vi "visualizeTDMS.vi"(8 "错误输入（无错误）":errorcluster) -> (0 "错误输出":errorcluster, 2 "强度图":dbl[][](graph), 3 "数据采集时间":string="2016/1/11 16:05:34")   [LabVIEW 2013]
panel:
  in  "save excel":bool
  out "file path out":path
  out "大小":i32
  out "数值":i32
  in  "确定按钮":bool
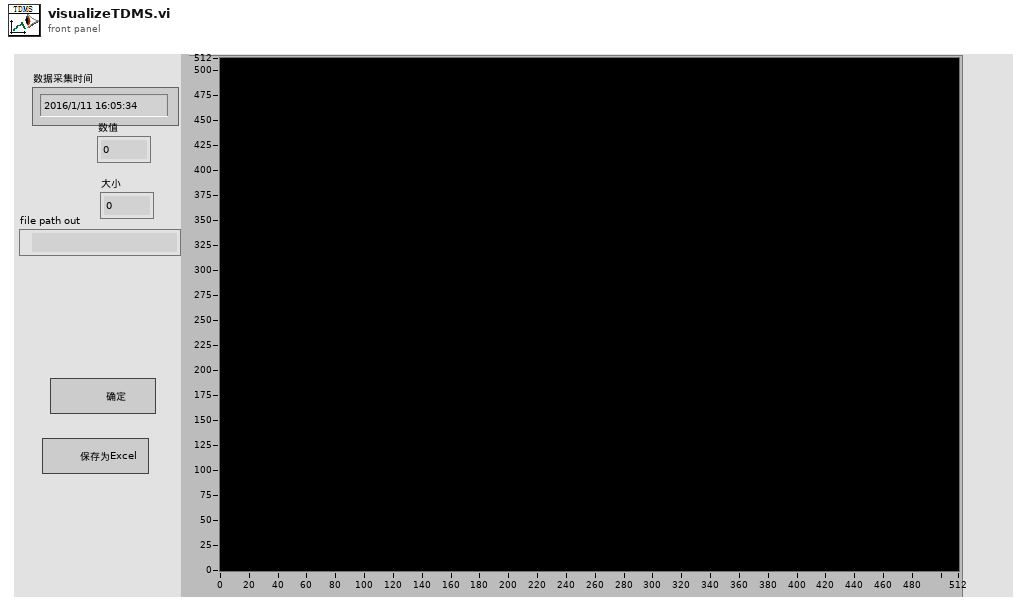
[diagram p1: front panel]
types:
  T1 = cluster{"Vx_Max":dbl, "Vy_Max":dbl, "Tx":dbl, "Row_N":i32, "Ratio":dbl}
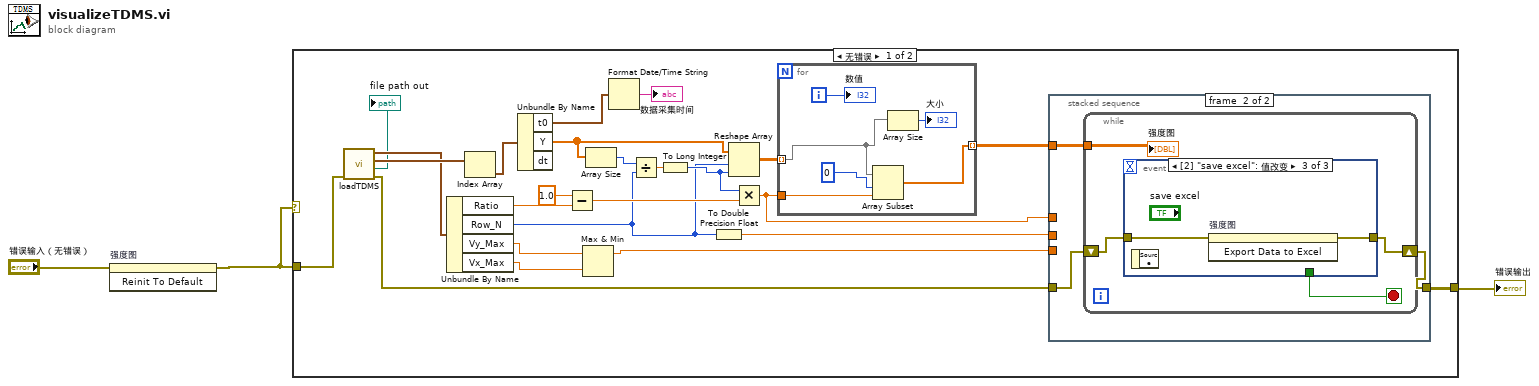
[diagram p0: block diagram]
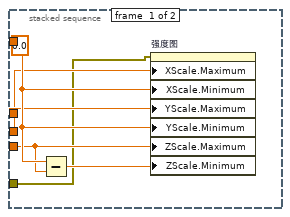
[diagram p2: hidden frame]
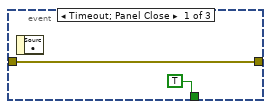
[diagram p3: hidden frame]
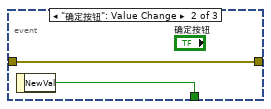
[diagram p4: hidden frame]
diagram:
  n1 = invoke on="强度图" class="IntGraph (严格)" method="Reinit To Default"(error in="错误输入（无错误）") -> (error out=w1:errorcluster)  [unwired: 2 in, 2 out]
  n2 = case shown="无错误" w1 {
    tunnel: w1 -> [w18 w53]
    tunnel: [w16 w53] -> w3
    frame No Error {
      n3 = call "loadTDMS.vi"("错误输入（无错误）"=w18) -> ("错误输出"=w17:errorcluster, "file path out"=→"file path out":path, "数据"=w27:waveform(dbl)[], "输出簇"=w15:T1)  [unwired: 7 in]
      n4 = Unbundle By Name(w15) -> ("Ratio"=w13:dbl, "Row_N"=w6:i32, "Vy_Max"=w21:dbl, "Vx_Max"=w20:dbl)
      n5 = Index Array(array=w27) -> (element=w26:waveform(dbl))  [unwired: 1 in]
      n6 = Unbundle By Name(w26) -> ("t0"=w25:timestamp, "Y"=w22:dbl[])  [unwired: 1 out]
      n7 = Subtract(x=1.0, y=w13) -> (x-y=w9:dbl)
      n8 = Max & Min(x=w21, y=w20) -> (max(x,y)=w19:dbl)  [unwired: 1 out]
      n9 = Array Size(array=w22) -> (size(s)=w23:i32)
      n10 = Format Date/Time String(seconds (now)=w25) -> (date/time string=→"数据采集时间":string)  [unwired: 2 in]
      n11 = Divide(x=w23, y=w6) -> (x/y=w10:dbl)
      n12 = To Long Integer(number=w10) -> (32bit integer=w8:i32)
      n13 = To Double Precision Float(number=w6) -> (double precision float=w5:dbl)
      n14 = Reshape Array(w22, w6, w8) -> (w14:dbl[][])
      n15 = Multiply(x=w8, y=w9) -> (x*y=w7:dbl)
      n16 = for {
        tunnel: w14 -> [w30] mode=indexing
        tunnel: [w29] -> w11 mode=indexing
        tunnel: w7 -> [w28]
        i -> [w33]
        n17 = Array Subset(array=w30, index=0 ("索引"), length=w28) -> (w29:dbl[])
        n18 = Array Size(array=w30) -> (size(s)=→"大小":i32)
        "数值" <- w33
      }
      n19 = stacked-sequence {
        tunnel: w11 -> [_ w42]
        tunnel: w5 -> [w35 _]
        tunnel: w19 -> [w37 _]
        tunnel: w17 -> [w34 w41]
        tunnel: [_ w40] -> w16
        tunnel: w7 -> [w36 _]
        frame #0 {
          w38 = 0.0
          n20 = Subtract(x=w38, y=w37) -> (x-y=w39:dbl)
          n21 = property on="强度图" class="IntGraph (严格)"(error in=w34, "XScale.Maximum"=w35, "XScale.Minimum"=w38, "YScale.Maximum"=w36, "YScale.Minimum"=w38, "ZScale.Maximum"=w37, "ZScale.Minimum"=w39) -> ()  [unwired: 1 in, 2 out]
        }
        frame #1 {
          n22 = while {
            tunnel: w42 -> [w45]
            shift-right: [w43] -> w40
            shift-left: w41 -> [w44]
            stop <- w46 stop-if-true
            n23 = event shown="[2] \"save excel\": 值改变" {
              selector: _ -> [_ _ _]
              dyn-events: _ -> [_ _ _]
              timeout: _ -> [_ _ _]
              tunnel: [TRUE w50 _] -> w46
              tunnel: w44 -> [w48 w49 w52]
              tunnel: [w48 w49 w51] -> w43
              event Timeout; Panel Close {
                n24 = event-data() -> ()  [unwired: 1 in, 1 out]
              }
              event "确定按钮": Value Change {
                n25 = event-data() -> ("NewVal"=w50:bool)  [unwired: 1 in]
              }
              event "save excel": Value Change {
                n26 = event-data() -> ()  [unwired: 1 in, 1 out]
                n27 = invoke on="强度图" class="IntGraph (严格)" method="Export Data to Excel"(error in=w52) -> (error out=w51:errorcluster)  [unwired: 2 in, 2 out]
              }
            }
            "强度图" <- w45
          }
        }
      }
    }
    frame Error {
    }
  }
  "错误输出" <- w3
